vi "1 Location to velocity.vi"(11 "Robot UTM Location":T2) -> (3 "Velocity":T1)   [LabVIEW 2011]
doc: "uses the low-pass differentiator to estimate velocity from a series of robot locations.\nTODO: does not deal with switches between UTM zones."
uses:
  2 Typedefs/UTM Location.ctl
  2 Typedefs/Velocity.ctl
  Low Pass Differentiator - DBL.vi
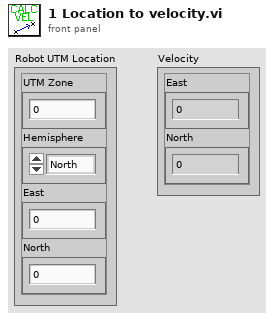
[diagram p1: front panel]
types:
  T1 = typedef "Velocity.ctl" = cluster{"East":dbl, "North":dbl}
  T2 = typedef "UTM Location.ctl" = cluster{"UTM Zone":dbl, "Hemisphere":enum16{"North", "South"}, "East":dbl, "North":dbl}
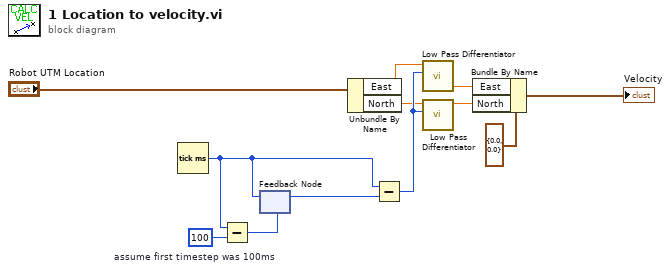
[diagram p0: block diagram]
diagram:
  w11 = u32 100  # assume first timestep was 100ms
  n1 = Tick Count (ms)() -> (millisecond timer value=w10:u32)
  n2 = Subtract(x=w10, y=w11) -> (x-y=w9:u32)
  n3 = feedback #1(w9) -> (w8:u32)
  n4 = feedback-in #1(w10) -> ()
  n5 = Unbundle By Name("Robot UTM Location") -> ("East"=w1:dbl, "North"=w2:dbl)
  n6 = Subtract(x=w10, y=w8) -> (x-y=w12:u32)
  n7 = call-poly "Low Pass Differentiator.vi"("dt"=w12, "X"=w1) -> ("dX, smoothed"=w4:dbl)  [unwired: 9 in]
  n8 = call-poly "Low Pass Differentiator.vi"("dt"=w12, "X"=w2) -> ("dX, smoothed"=w3:dbl)  [unwired: 9 in]
  n9 = Bundle By Name(cluster=T1 {"East"=0.0, "North"=0.0} ("Velocity 2"), "East"=w4, "North"=w3) -> (→"Velocity":T1)
